vi "Drop unmatched VCluster data.vi"(8 "error in (no error)":errorcluster, 10 "Columns":string[](array[string]), 11 "VCluster in":variant) -> (0 "error out":errorcluster, 2 "VCluster Columns":string[](array[string]), 3 "VCluster out":variant)   [LabVIEW 2020, in "Database Reuse.lvlib"]
uses:
  Database Reuse.lvlib
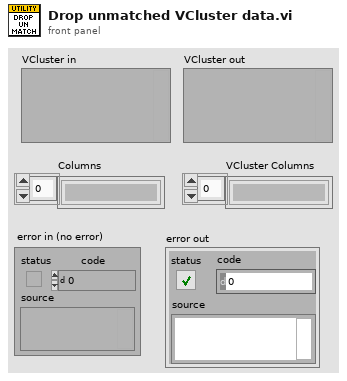
[diagram p1: front panel]
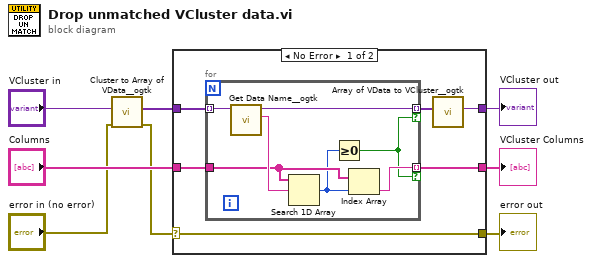
[diagram p0: block diagram]
diagram:
  n1 = call <userlib>:"Cluster to Array of VData__ogtk.vi"("error in (no error)"="error in (no error)", "Cluster"="VCluster in") -> ("error out"=w1:errorcluster, "Array of VData"=w4:variant[])  [unwired: 8 in]
  n2 = case shown="No Error" w1 {
    selector: w1 -> [w11 w22]
    tunnel: [w14 _] -> w8
    tunnel: "Columns" -> [w13 _]
    tunnel: w4 -> [w12 _]
    tunnel: [w11 w22] -> w6
    tunnel: [w9 _] -> w5
    frame No Error {
      n3 = for {
        tunnel: w12 -> [w16] mode=indexing
        tunnel: w13 -> [w20]
        tunnel: [w18] -> w10 mode=indexing if=w15
        tunnel: [w17] -> w14 mode=indexing if=w15
        n4 = call <userlib>:"Get Data Name__ogtk.vi"("Data"=w16) -> ("Data Name"=w21:string, "Data dup"=w18:variant)  [unwired: 8 in, 1 out]
        n5 = Search 1D Array(1D array=w20, element=w21) -> (index of element=w19:i32)  [unwired: 1 in]
        n6 = Greater Or Equal To 0?(x=w19) -> (x >= 0?=w15:bool)
        n7 = Index Array(array=w20, index=w19) -> (element=w17:string)
      }
      n8 = call <userlib>:"Array of VData to VCluster__ogtk.vi"("Array"=w10) -> ("VCluster"=w9:variant)  [unwired: 9 in, 1 out]
    }
    frame Error {
    }
  }
  "VCluster out" <- w5
  "VCluster Columns" <- w8
  "error out" <- w6
